vi "StringsToEnergy(SI)_Ophir.vi"(8 "error in":errorcluster, 10 "input string":string) -> (0 "error out":errorcluster, 2 "Energy/Power(SI)":dbl)   [LabVIEW 2011]
uses:
  <vilib>/regexp/Match Regular Expression.xnode
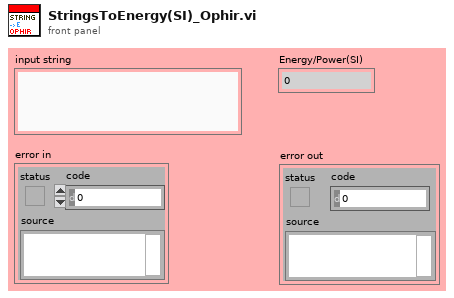
[diagram p1: front panel]
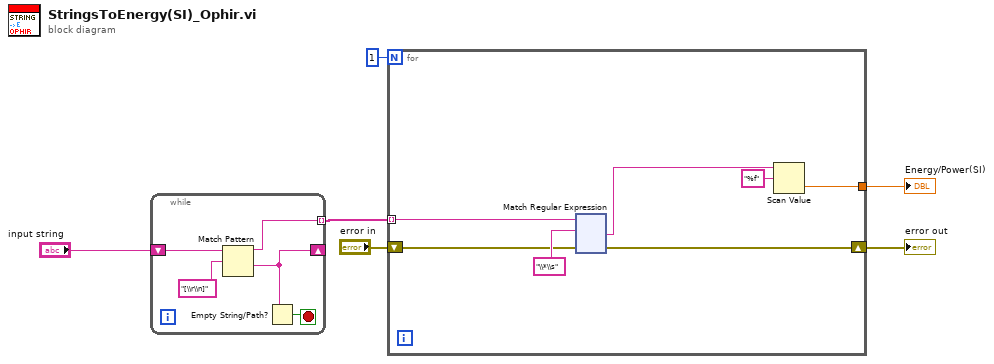
[diagram p0: block diagram]
diagram:
  n1 = while {
    tunnel: [w9] -> w5 mode=indexing
    shift-right: [w7] -> _
    shift-left: "input string" -> [w11]
    stop <- w8 stop-if-true
    n2 = Match Pattern(string=w11, regular expression="[\\r\\n]") -> (before substring=w9:string, after substring=w7:string)  [unwired: 1 in, 2 out]
    n3 = Empty String/Path?(string/path=w7) -> (empty?=w8:bool)
  }
  n4 = for {
    N: 1 -> [_]
    tunnel: w5 -> [w17] mode=indexing
    shift-right: [w12] -> w3
    shift-left: "error in" -> [w16]
    tunnel: [w14] -> w1
    n5 = xnode "Match Regular Expression"("input string"=w17, "regular expression"="\\*\\s", "error in"=w16) -> ("after match"=w13:string, "error out"=w12:errorcluster)  [unwired: 3 in, 3 out]
    n6 = Scan Value(string=w13, format string="%f") -> (value=w14:dbl)  [unwired: 1 in, 1 out]
  }
  "error out" <- w3
  "Energy/Power(SI)" <- w1
